vi "UHR-Fleezers Control (host) - Lorentz v2.vi"() -> ()   [LabVIEW 2014] (continued)
            n1300 = To Word Integer(number=w1984) -> (16bit integer=w1982:cluster{"Set 1":i16, "Set 2":i16})
          }
          frame True {
            n1301 = Unbundle By Name(w1992) -> ("Set 1"=w1991:dbl, "Set 2"=w1990:dbl)
            n1302 = Unbundle By Name(w1998) -> ("Set 1"=w1997:dbl, "Set 2"=w1996:dbl)
            n1303 = Unbundle By Name(w1995) -> ("Set 1"=w1994:bool, "Set 2"=w1993:bool)
            n1304 = Select(t=w1991, s=w1994, f=w1997) -> (s? t:f=w1989:dbl)
            n1305 = Select(t=w1990, s=w1993, f=w1996) -> (s? t:f=w1988:dbl)
            n1306 = Bundle By Name(cluster=w1998, "Set 1"=w1989, "Set 2"=w1988) -> (w1986:cluster{"Set 1":dbl, "Set 2":dbl})
            n1307 = local write "Setpoints (V)"(w1986) -> ()
            n1308 = Multiply(x=3276.7, y=w1986) -> (x*y=w1987:cluster{"Set 1":dbl, "Set 2":dbl})
            n1309 = To Word Integer(number=w1987) -> (16bit integer=w1999:cluster{"Set 1":i16, "Set 2":i16})
          }
        }
        n1310 = Unbundle By Name(w1971) -> ("Set 1"=w1970:i16, "Set 2"=w1969:i16)
        n1311 = xnode "Read/Write Control"("FPGA VI Reference In"=w1968, "error in"=w1967, "FB Setpoint Set 1"=w1970, "FB Setpoint Set 2"=w1969) -> ("error out"=w1966:errorcluster)  [unwired: 1 out]
      }
      event "+ phase (GI)", "- phase (GI)", "+ phase (GI) 2", "- phase (GI) 2", "+ phase (RI)", "- phase (RI)", "+ phase (Green FB)", "- phase (Green FB)", "- phase (BI AO)", "+ phase (BI AO)", "- phase (BI DO)", "+ phase (BI DO)": Value Change {
        n1312 = event-data() -> ()  [unwired: 7 out]
        n1313 = Or(x="+ phase (GI)", y="- phase (GI)") -> (x .or. y?=w2035:bool)
        n1314 = Negate(x="Phase adj. (GI)") -> (-x=w2040:i16)
        n1315 = Select(t=w2040, s="+ phase (GI)", f="Phase adj. (GI)") -> (s? t:f=w2039:i16)
        n1316 = Or(x="+ phase (GI) 2", y="- phase (GI) 2") -> (x .or. y?=w2026:bool)
        n1317 = Negate(x="Phase adj. (GI) 2") -> (-x=w2031:i16)
        n1318 = Select(t=w2031, s="+ phase (GI) 2", f="Phase adj. (GI) 2") -> (s? t:f=w2027:i16)
        n1319 = Negate(x="Phase adj. (RI)") -> (-x=w2025:i16)
        n1320 = Or(x="+ phase (RI)", y="- phase (RI)") -> (x .or. y?=w2021:bool)
        n1321 = Select(t=w2025, s="+ phase (RI)", f="Phase adj. (RI)") -> (s? t:f=w2020:i16)
        n1322 = Or(x="+ phase (Green FB)", y="- phase (Green FB)") -> (x .or. y?=w2014:bool)
        n1323 = Negate(x="Phase adj. (Green FB)") -> (-x=w2019:i16)
        n1324 = Select(t=w2019, s="+ phase (Green FB)", f="Phase adj. (Green FB)") -> (s? t:f=w2015:i16)
        n1325 = Negate(x="Phase adj. (BI AO)") -> (-x=w2013:i16)
        n1326 = Or(x="+ phase (BI AO)", y="- phase (BI AO)") -> (x .or. y?=w2003:bool)
        n1327 = Select(t=w2013, s="+ phase (BI AO)", f="Phase adj. (BI AO)") -> (s? t:f=w2005:i16)
        n1328 = Negate(x="Phase adj. (BI DO)") -> (-x=w2009:i16)
        n1329 = Or(x="+ phase (BI DO)", y="- phase (BI DO)") -> (x .or. y?=w2002:bool)
        n1330 = Select(t=w2009, s="+ phase (BI DO)", f="Phase adj. (BI DO)") -> (s? t:f=w2004:i16)
        n1331 = xnode "Read/Write Control"("FPGA VI Reference In"=w2001, "Phase count adjustment (GI)"=w2039, "Phase count adjustment (GI) 2"=w2027, "Phase count adjustment (RI)"=w2020, "Phase count adjustment (Green FB)"=w2015, "Phase count adjustment (BI AO)"=w2005, "Phase count adjustment (BI D)"=w2004) -> ("FPGA VI Reference Out"=w2037:T31, "error out"=w2038:errorcluster)  [unwired: 1 in]
        n1332 = xnode "Read/Write Control"("FPGA VI Reference In"=w2037, "error in"=w2038, "+ phase (GI)"=w2035, "+ phase (GI) 2"=w2026, "+ phase (RI)"=w2021, "+ phase (Green FB)"=w2014, "+ phase (BI AO)"=w2003, "+ phase (BI D)"=w2002) -> ("error out"=w2036:errorcluster)  [unwired: 1 out]
      }
      event "Green Laser ON/OFF", "Red Laser ON/OFF", "Blue Laser ON/OFF": Value Change {
        # "This loop shouldn't be initialized.  The main 'laser ON' settings should dominate and set the others."
        n1333 = event-data() -> ()  [unwired: 7 out]
        n1334 = property on="Red Laser ON" class="Bool (strict)"("Val(Sgnl)"="Red Laser ON/OFF") -> ()  [unwired: 2 in, 2 out]
        n1335 = property on="Blue Laser ON" class="Bool (strict)"("Val(Sgnl)"="Blue Laser ON/OFF") -> ()  [unwired: 2 in, 2 out]
        n1336 = property on="Green Laser ON" class="Bool (strict)"("Val(Sgnl)"="Green Laser ON/OFF") -> ()  [unwired: 2 in, 2 out]
      }
      event "Laser interlacing mode", "Green Laser ON", "Red Laser ON", "Blue Laser ON": Value Change {
        n1337 = event-data() -> ()  [unwired: 7 out]
        n1338 = local write "Green Laser ON/OFF"("Green Laser ON") -> ()
        n1339 = local write "Blue Laser ON/OFF"("Blue Laser ON") -> ()
        n1340 = local write "Red Laser ON/OFF"("Red Laser ON") -> ()
        n1341 = case shown="False" "Green Laser ON" {
          tunnel: "Laser interlacing mode" -> [_ w2101]
          tunnel: [enum32{"Laser ON", "Laser OFF", "Interlace"}."Laser OFF" ("Green laser mode") w2101] -> w2077
          tunnel: [FALSE w2097] -> w2076
          frame False {
          }
          frame True {
            n1342 = local read "Green FB On/Off"() -> (w2098:bool)
            n1343 = Equal?(x=w2101, y=enum32{"Laser ON", "Laser OFF", "Interlace"}."Interlace") -> (x = y?=w2099:bool)
            n1344 = And(x=w2099, y=w2098) -> (x .and. y?=w2097:bool)
          }
        }
        n1345 = case shown="True" "Red Laser ON" {
          tunnel: "Laser interlacing mode" -> [_ w2094]
          tunnel: [enum32{"Laser ON", "Laser OFF", "Interlace"}."Laser OFF" ("Green laser mode") w2094] -> w2073
          tunnel: [FALSE w2090] -> w2072
          frame False {
          }
          frame True {
            n1346 = local read "Red FB On/Off"() -> (w2091:bool)
            n1347 = Equal?(x=w2094, y=enum32{"Laser ON", "Laser OFF", "Interlace"}."Interlace") -> (x = y?=w2092:bool)
            n1348 = And(x=w2092, y=w2091) -> (x .and. y?=w2090:bool)
          }
        }
        n1349 = case shown="True" "Blue Laser ON" {
          tunnel: "Laser interlacing mode" -> [_ w2085]
          tunnel: [enum32{"Laser ON", "Laser OFF", "Interlace"}."Laser OFF" ("Green laser mode") w2085] -> w2069
          tunnel: [FALSE w2083] -> w2068
          frame False {
          }
          frame True {
            n1350 = local read "Blue FB On/Off"() -> (w2084:bool)
            n1351 = Equal?(x=w2085, y=enum32{"Laser ON", "Laser OFF", "Interlace"}."Interlace") -> (x = y?=w2086:bool)
            n1352 = And(x=w2086, y=w2084) -> (x .and. y?=w2083:bool)
          }
        }
        n1353 = xnode "Read/Write Control"("FPGA VI Reference In"=w2067, "Operating Mode"=w2077, "Operating Mode 2"=w2077, "Green FB On/Off"=w2076, "Red Laser Operating Mode"=w2073, "RI Operating Mode 2"=w2073, "Red FB On/Off"=w2072, "BI Operating Mode (AO)"=w2069, "Blue Laser Operating Mode (D)"=w2069, "Blue FB On/Off"=w2068) -> ("error out"=w2078:errorcluster)  [unwired: 1 in, 1 out]
        n1354 = local read "Red FB On/Off"() -> (w2050:bool)
        n1355 = local read "Green FB On/Off"() -> (w2052:bool)
        n1356 = local read "Green Laser ON"() -> (w2051:bool)
        n1357 = local read "Red Laser ON"() -> (w2049:bool)
        n1358 = And(x=w2050, y=w2049) -> (x .and. y?=w2055:bool)
        n1359 = And(x=w2052, y=w2051) -> (x .and. y?=w2061:bool)
        n1360 = local read "Red laser intensity (V)"() -> (w2054:dbl)
        n1361 = local read "Red FB Setpoint (mV)"() -> (w2053:dbl)
        n1362 = local read "Green FB Setpoint (mV)"() -> (w2064:dbl)
        n1363 = local read "Green laser intensity (V)"() -> (w2066:dbl)
        n1364 = Multiply(x=w2054, y=1000.0) -> (x*y=w2058:dbl)
        n1365 = Subtract(x=w2053, y=5.0) -> (x-y=w2057:dbl)
        n1366 = Multiply(x=w2066, y=1000.0) -> (x*y=w2063:dbl)
        n1367 = Subtract(x=w2064, y=5.0) -> (x-y=w2062:dbl)
        n1368 = Less Or Equal?(x=w2058, y=w2057) -> (x <= y?=w2056:bool)
        n1369 = Less Or Equal?(x=w2063, y=w2062) -> (x <= y?=w2060:bool)
        n1370 = And(x=w2055, y=w2056) -> (x .and. y?=w2045:bool)
        n1371 = And(x=w2061, y=w2060) -> (x .and. y?=w2046:bool)
        n1372 = Or(x=w2046, y=w2045) -> (x .or. y?=w2044:bool)
        n1373 = case shown="True" w2044 {
          frame False {
            n1374 = local write "Laser Intensity Low (bugs to fix)"(FALSE ("Laser Intensity Low")) -> ()
          }
          frame True {
            n1375 = local write "Laser Intensity Low (bugs to fix)"(TRUE ("Laser Intensity Low")) -> ()
          }
        }
      }
      event "Invert laser interlacing": Value Change {
        n1376 = event-data() -> ()  [unwired: 7 out]
        n1377 = xnode "Read/Write Control"("FPGA VI Reference In"=w2102, "Invert GI"="Invert laser interlacing", "Invert GI 2"="Invert laser interlacing", "Invert RI"="Invert laser interlacing", "Invert RI 2"="Invert laser interlacing", "Invert BI (AO)"="Invert laser interlacing", "Invert BI (D)"="Invert laser interlacing") -> ("error out"=w2104:errorcluster)  [unwired: 1 in, 1 out]
      }
      event "Green FB Setpoint (mV)", "Green FB Gains", "Green FB On/Off", "Green Intensity % (FB OFF)", "Green int current ON count adj": Value Change {
        n1378 = event-data() -> ()  [unwired: 7 out]
        n1379 = local read "Green FB Setpoint (mV)"() -> (w2124:dbl)
        n1380 = Multiply(x=w2124, y=3.2767) -> (x*y=w2123:dbl)
        n1381 = local read "Green Intensity % (FB OFF)"() -> (w2127:dbl)
        n1382 = Multiply(x=w2127, y=655.35) -> (x*y=w2128:dbl)
        n1383 = To Unsigned Word Integer(number=w2128) -> (unsigned 16bit integer=w2126:u16)
        n1384 = local read "Green int current ON count adj"() -> (w2130:u32)
        n1385 = local read "Laser interlacing mode"() -> (w2121:enum32{"Laser ON", "Laser OFF", "Interlace"})
        n1386 = local read "Green FB Gains"() -> (w2118:T11)
        n1387 = local read "Green Laser ON"() -> (w2122:bool)
        n1388 = local read "Green FB On/Off"() -> (w2131:bool)
        n1389 = Equal?(x=w2121, y=enum32{"Laser ON", "Laser OFF", "Interlace"}."Interlace") -> (x = y?=w2119:bool)
        n1390 = Unbundle By Name(w2118) -> ("proportional gain (Kc)"=w2117:i16, "integral gain (Kc*Ts/Ti)"=w2116:i16, "derivative gain (Kc*Td/Ts)"=w2115:i16)
        n1391 = Compound Arithmetic op=AND(w2119, w2131, w2122) -> (w2105:bool)
        n1392 = local read "Green FB Setpoint (mV)"() -> (w2109:dbl)
        n1393 = local read "Green laser intensity (V)"() -> (w2112:dbl)
        n1394 = xnode "Read/Write Control"("FPGA VI Reference In"=w2114, "Green FB Setpoint"=w2123, "Green FB On/Off"=w2105, "Current Out"=w2126, "Green int current ON count adj"=w2130, "P3"=w2117, "I3"=w2116, "D3"=w2115) -> ("error out"=w2132:errorcluster)  [unwired: 1 in, 1 out]
        n1395 = Multiply(x=w2112, y=1000.0) -> (x*y=w2108:dbl)
        n1396 = Subtract(x=w2109, y=5.0) -> (x-y=w2107:dbl)
        n1397 = Less Or Equal?(x=w2108, y=w2107) -> (x <= y?=w2106:bool)
        n1398 = And(x=w2105, y=w2106) -> (x .and. y?=w2113:bool)
        n1399 = case shown="True" w2113 {
          frame False {
            n1400 = local write "Laser Intensity Low (bugs to fix)"(FALSE ("Laser Intensity Low")) -> ()
          }
          frame True {
            n1401 = local write "Laser Intensity Low (bugs to fix)"(TRUE ("Laser Intensity Low")) -> ()
          }
        }
      }
      event "Blue FB Setpoint (mV)", "Blue FB Gains", "Blue FB On/Off", "Blue Intensity % (FB OFF)", "Blue int AO ON count adjust": Value Change {
        # "Triggers blue laser serial command"
        # "16 bit analog out"
        n1402 = event-data() -> ()  [unwired: 7 out]
        n1403 = Multiply(x="Blue FB Setpoint (mV)", y=3.2767) -> (x*y=w2152:dbl)
        n1404 = Multiply(x="Blue Intensity % (FB OFF)", y=0.8) -> (x*y=w2135:dbl)
        n1405 = Number To Decimal String(number=w2135) -> (decimal integer string=w2136:string)  [unwired: 1 in]
        n1406 = Multiply(x="Blue Intensity % (FB OFF)", y=655.35) -> (x*y=w2155:dbl)
        n1407 = local write "Blue Laser Power (mW)\n(Constant Power Mode)"(w2136) -> ()
        n1408 = To Unsigned Word Integer(number=w2155) -> (unsigned 16bit integer=w2154:u16)
        n1409 = local read "Laser interlacing mode"() -> (w2150:enum32{"Laser ON", "Laser OFF", "Interlace"})
        n1410 = Unbundle By Name("Blue FB Gains") -> ("proportional gain (Kc)"=w2147:i16, "integral gain (Kc*Ts/Ti)"=w2146:i16, "derivative gain (Kc*Td/Ts)"=w2145:i16)
        n1411 = local read "Blue Laser ON"() -> (w2140:bool)
        n1412 = Equal?(x=w2150, y=enum32{"Laser ON", "Laser OFF", "Interlace"}."Interlace") -> (x = y?=w2148:bool)
        n1413 = Compound Arithmetic op=AND(w2148, "Blue FB On/Off", w2140) -> (w2151:bool)
        n1414 = xnode "Read/Write Control"("FPGA VI Reference In"=w2139, "Blue FB Setpoint"=w2152, "Blue FB On/Off"=w2151, "BI Current Out"=w2154, "Blue current ON count adj (AO)"="Blue int AO ON count adjust", "P5"=w2147, "I5"=w2146, "D5"=w2145) -> ("error out"=w2157:errorcluster)  [unwired: 1 in, 1 out]
      }
      event "Red FB Setpoint (mV)", "Red FB Gains", "Red FB On/Off", "Red Intensity % (FB OFF)": Value Change {
        n1415 = event-data() -> ()  [unwired: 7 out]
        n1416 = local read "Red FB Setpoint (mV)"() -> (w2178:dbl)
        n1417 = Multiply(x=w2178, y=3.2767) -> (x*y=w2177:dbl)
        n1418 = local read "Red Intensity % (FB OFF)"() -> (w2168:dbl)
        n1419 = Multiply(x=w2168, y=655.35) -> (x*y=w2181:dbl)
        n1420 = To Unsigned Word Integer(number=w2181) -> (unsigned 16bit integer=w2180:u16)
        n1421 = local read "Laser interlacing mode"() -> (w2175:enum32{"Laser ON", "Laser OFF", "Interlace"})
        n1422 = local read "Red FB Gains"() -> (w2172:T11)
        n1423 = local read "Red Laser ON"() -> (w2176:bool)
        n1424 = local read "Red FB On/Off"() -> (w2183:bool)
        n1425 = Equal?(x=w2175, y=enum32{"Laser ON", "Laser OFF", "Interlace"}."Interlace") -> (x = y?=w2173:bool)
        n1426 = Unbundle By Name(w2172) -> ("proportional gain (Kc)"=w2171:i16, "integral gain (Kc*Ts/Ti)"=w2170:i16, "derivative gain (Kc*Td/Ts)"=w2169:i16)
        n1427 = Compound Arithmetic op=AND(w2173, w2183, w2176) -> (w2160:bool)
        n1428 = local read "Red laser intensity (V)"() -> (w2159:dbl)
        n1429 = local read "Red FB Setpoint (mV)"() -> (w2158:dbl)
        n1430 = xnode "Read/Write Control"("FPGA VI Reference In"=w2167, "Red FB Setpoint"=w2177, "Red FB On/Off"=w2160, "RI Current Out"=w2180, "P4"=w2171, "I4"=w2170, "D4"=w2169) -> ("error out"=w2184:errorcluster)  [unwired: 1 in, 1 out]
        n1431 = Multiply(x=w2159, y=1000.0) -> (x*y=w2164:dbl)
        n1432 = Subtract(x=w2158, y=5.0) -> (x-y=w2163:dbl)
        n1433 = Less Or Equal?(x=w2164, y=w2163) -> (x <= y?=w2162:bool)
        n1434 = And(x=w2160, y=w2162) -> (x .and. y?=w2161:bool)
        n1435 = case shown="False" w2161 {
          frame False {
            n1436 = local write "Laser Intensity Low (bugs to fix)"(FALSE ("Laser Intensity Low")) -> ()
          }
          frame True {
            n1437 = local write "Laser Intensity Low (bugs to fix)"(TRUE ("Laser Intensity Low")) -> ()
          }
        }
      }
      event "+ phase (APD 1 Gate)", "- phase (APD 1 Gate)", "+ phase (APD 2 Gate)", "- phase (APD 2 Gate)", "+ phase (APD 3 Gate)", "- phase (APD 3 Gate)", "+ phase (APD Acq)", "- phase (APD Acq)": Value Change {
        n1438 = event-data() -> ()  [unwired: 7 out]
        n1439 = local read "Phase Adj. (APD 1 Gate)"() -> (w2207:i16)
        n1440 = Or(x="- phase (APD 1 Gate)", y="+ phase (APD 1 Gate)") -> (x .or. y?=w2209:bool)
        n1441 = Negate(x=w2207) -> (-x=w2214:i16)
        n1442 = Select(t=w2214, s="+ phase (APD 1 Gate)", f=w2207) -> (s? t:f=w2213:i16)
        n1443 = local read "Phase Adj. (APD 2 Gate)"() -> (w2204:i16)
        n1444 = Or(x="- phase (APD 2 Gate)", y="+ phase (APD 2 Gate)") -> (x .or. y?=w2202:bool)
        n1445 = Negate(x=w2204) -> (-x=w2206:i16)
        n1446 = Select(t=w2206, s="+ phase (APD 2 Gate)", f=w2204) -> (s? t:f=w2203:i16)
        n1447 = Negate(x="Phase Adj. (APD 3 Gate)") -> (-x=w2201:i16)
        n1448 = Or(x="- phase (APD 3 Gate)", y="+ phase (APD 3 Gate)") -> (x .or. y?=w2197:bool)
        n1449 = Select(t=w2201, s="+ phase (APD 3 Gate)", f="Phase Adj. (APD 3 Gate)") -> (s? t:f=w2198:i16)
        n1450 = local read "Phase Adj. (APD Acq)"() -> (w2195:i16)
        n1451 = Or(x="- phase (APD Acq)", y="+ phase (APD Acq)") -> (x .or. y?=w2193:bool)
        n1452 = Negate(x=w2195) -> (-x=w2196:i16)
        n1453 = Select(t=w2196, s="+ phase (APD Acq)", f=w2195) -> (s? t:f=w2194:i16)
        n1454 = xnode "Read/Write Control"("FPGA VI Reference In"=w2187, "Phase count adjustment (APD 1 Gate)"=w2213, "Phase count adjustment (APD 2 Gate)"=w2203, "Phase count adjustment (APD 3 Gate)"=w2198, "Phase Count Adjustment (APD Acq)"=w2194) -> ("FPGA VI Reference Out"=w2211:T31, "error out"=w2212:errorcluster)  [unwired: 1 in]
        n1455 = xnode "Read/Write Control"("FPGA VI Reference In"=w2211, "error in"=w2212, "+ phase (APD 1 Gate)"=w2209, "+ phase (APD 2 Gate)"=w2202, "+ phase (APD 3 Gate)"=w2197, "+ phase (APD Acq)"=w2193) -> ("error out"=w2210:errorcluster)  [unwired: 1 out]
      }
      event "Invert APD Gate", "APD Gate ON Count", "APD Gate OFF Count", "APD Gate", "APD Integration Time (s)", "APD AO Scale Factor", "Duty Frequency (ON 1/N cycles)", "Interlace ON count", "Interlace OFF count": Value Change {
        n1456 = event-data() -> ()  [unwired: 7 out]
        n1457 = Add(x="Interlace ON count", y="Interlace OFF count") -> (x+y=w2221:u16)
        n1458 = Add(x="APD Gate ON Count", y="APD Gate OFF Count") -> (x+y=w2232:u16)
        n1459 = Multiply(x="Duty Frequency (ON 1/N cycles)", y=w2221) -> (x*y=w2217:u16)
        "Green AI Count" <- w2217
        "Red AI Count" <- w2217
        "Blue AI Count" <- w2217
        n1460 = Subtract(x=w2217, y="Interlace ON count") -> (x-y=w2220:u16)
        n1461 = Multiply(x=w2232, y="Duty Frequency (ON 1/N cycles)") -> (x*y=w2231:u16)
        n1462 = Subtract(x=w2231, y="APD Gate ON Count") -> (x-y=w2230:u16)
        n1463 = local read "DMA Update Period (s)"() -> (w2233:dbl)
        n1464 = Multiply(x="APD Integration Time (s)", y=40000000.0) -> (x*y=w2237:dbl)
        n1465 = Reciprocal(x="APD Integration Time (s)") -> (1/x=→"APD Acq Rate (Hz)":dbl)
        n1466 = To Unsigned Long Integer(number=w2237) -> (unsigned 32bit integer=w2223:u32)
        "APD Int. Count" <- w2223
        n1467 = local read "Number of APDs"() -> (w2216:u8)
        n1468 = Divide(x=w2233, y="APD Integration Time (s)") -> (x/y=w2235:dbl)
        n1469 = Multiply(x=w2216, y=w2235) -> (x*y=w2234:dbl)
        n1470 = local write "APD Samples/FIFO Acq."(w2235) -> ()
        n1471 = local write "APD Elements/DMA read"(w2234) -> ()
        n1472 = xnode "Read/Write Control"("FPGA VI Reference In"=w2215, "Invert APD Gate"="Invert APD Gate", "APD Gate ON Count"="APD Gate ON Count", "APD Gate OFF Count"=w2230, "APD Acq Rate Count"=w2223, "APD Gate Operating Mode"="APD Gate", "APD AO scale factor"="APD AO Scale Factor", "Green interlace ON count"="Interlace ON count", "Green interlace OFF count"=w2220, "Green interlace ON count 2"="Interlace ON count", "Green interlace OFF count 2"=w2220, "Green FB Count"=w2217, "Red interlace ON count"="Interlace ON count", "Red interlace OFF count"="Interlace OFF count", "Blue ON count (AO)"="Interlace ON count", "Blue OFF count (AO)"="Interlace OFF count", "Blue interlace OFF count (D)"="Interlace OFF count", "Blue interlace ON count (D)"="Interlace ON count") -> ("error out"=w2239:errorcluster)  [unwired: 1 in, 1 out]
      }
      event "Neg. TTrig FPGA": Value Change {
        n1473 = event-data() -> ()  [unwired: 7 out]
        n1474 = xnode "Read/Write Control"("FPGA VI Reference In"=w2240, "TTrig Negate Pos"="Neg. TTrig FPGA") -> ()  [unwired: 1 in, 2 out]
      }
      event "Test ttrig": Value Change {
        n1475 = event-data() -> ()  [unwired: 7 out]
        n1476 = xnode "Read/Write Control"("FPGA VI Reference In"=w2242, "TTrig?"=TRUE) -> ("error out"=w2244:errorcluster)  [unwired: 1 in, 1 out]
      }
      event "Number of F/B Scans (AOD)", "Scan Speed (nm/s)", "Scan BD", "Initial delta (MHz)", "Step Size (nm)", "Scan Range (nm)": Value Change {
        w2308 = 123.0  # AOM cal (nm/MHz)
        n1477 = event-data() -> ()  [unwired: 7 out]
        n1478 = local read "BD 1 Frequency 1 (MHz)"() -> (w2291:dbl)
        n1479 = local read "AOM X Cal (nm/MHz)"() -> (w2283:dbl)
        n1480 = local read "X RF Frequency Limits (MHz)"() -> (w2295:T20)
        n1481 = local read "Y RF Frequency Limits (MHz)"() -> (w2292:T20)
        n1482 = local read "BD 2 Frequency 1 (MHz)"() -> (w2297:dbl)
        n1483 = Negate(x="Scan Range (nm)") -> (-x=w2261:dbl)
        n1484 = Divide(x=w2261, y=w2283) -> (x/y=w2265:dbl)
        n1485 = Select(t=w2295, s="Scan BD", f=w2292) -> (s? t:f=w2294:T20)
        n1486 = Select(t=w2291, s="Scan BD", f=w2297) -> (s? t:f=w2296:dbl)
        n1487 = Unbundle By Name(w2294) -> ("Maximum"=w2303:dbl, "Minimum"=w2302:dbl)
        n1488 = Add(x=w2265, y=w2296) -> (x+y=w2300:dbl)
        n1489 = Divide(x=w2261, y="Step Size (nm)") -> (x/y=w2280:dbl)
        n1490 = Divide(x="Step Size (nm)", y=w2283) -> (x/y=w2289:dbl)
        n1491 = Absolute Value(x=w2280) -> (abs(x)=w2264:dbl)
        n1492 = Sign(1:w2261) -> (0:w2262:dbl)
        n1493 = In Range and Coerce(upper limit=w2303, x=w2300, lower limit=w2302) -> (coerced(x)=w2299:dbl, In Range?=w2301:bool)
        n1494 = To Unsigned Quad Integer(1:w2264) -> (0:w2279:u64)
        "Scan steps (AOD)" <- w2279
        n1495 = call "IR AOM freq to word.vi"("Frequency In (MHz)"=w2289) -> ("Frequency Word Out (double)"=w2286:dbl)
        n1496 = Multiply(x=w2262, y=w2286) -> (x*y=w2263:dbl)
        n1497 = Subtract(x=w2300, y=w2299) -> (x-y=w2298:dbl)
        n1498 = To Quad Integer(1:w2263) -> (0:w2285:i64)
        "Incr. int (AOD)" <- w2285
        n1499 = Subtract(x=w2265, y=w2298) -> (x-y=w2284:dbl)
        "Scan Range (MHz)" <- w2284
        n1500 = Select(t=w2265, s=w2301, f=w2284) -> (s? t:f=w2304:dbl)
        n1501 = Multiply(x=w2284, y=w2283) -> (x*y=w2282:dbl)
        n1502 = Decrement(x=w2279) -> (x-1=w2332:u64)
        n1503 = Negate(x=w2282) -> (-x=w2278:dbl)
        n1504 = local write "Scan Range (nm)"(w2278) -> ()
        n1505 = Divide(x=w2304, y=w2332) -> (x/y=w2288:dbl)
        "Scan Increment (MHz)" <- w2288
        n1506 = call "IR AOM freq to word.vi"("Frequency In (MHz)"=w2288) -> ("Frequency Word Out (double)"=w2287:dbl)
        n1507 = Divide(x="Step Size (nm)", y="Scan Speed (nm/s)") -> (x/y=w2275:dbl)
        n1508 = To Quad Integer(1:w2287) -> ()  [unwired: 1 out]
        n1509 = local read "Number Interlace Sets"() -> (w2259:u8)
        n1510 = local read "AI Count (ticks)"() -> (w2260:u16)
        n1511 = local read "Total Counts (ticks)"() -> (w2258:u16)
        n1512 = local read "# Samples/trap"() -> (w2290:u32)
        n1513 = Multiply(x=w2260, y=w2259) -> (x*y=w2257:u16)
        n1514 = Divide(x=w2258, y=w2257) -> (x/y=w2256:dbl)
        n1515 = Select(t=w2291, s="Scan BD", f=w2297) -> (s? t:f=w2329:dbl)
        "Initial freq. (MHz)" <- w2329
        n1516 = Add(x=w2304, y=w2329) -> (x+y=→"Final freq. (MHz)":dbl)
        n1517 = Divide(x=w2258, y=40000000.0) -> (x/y=w2274:dbl)
        n1518 = Divide(x=w2275, y=w2274) -> (x/y=w2273:dbl)
        n1519 = To Unsigned Quad Integer(1:w2273) -> (0:w2248:u64)
        n1520 = Quotient & Remainder(x=w2248, y=u64 2) -> (x-y*floor(x/y)=w2252:u64)  [unwired: 1 out]
        n1521 = Equal?(x=w2252, y=u64 0) -> (x = y?=w2250:bool)
        n1522 = Decrement(x=w2248) -> (x-1=w2249:u64)
        n1523 = Select(t=w2248, s=w2250, f=w2249) -> (s? t:f=w2247:u64)
        "Cycles/step (AOD)" <- w2247
        n1524 = xnode "Read/Write Control"("FPGA VI Reference In"=w2246, "Scan steps"=w2279, "Number of scans"="Number of F/B Scans (AOD)", "Cycles per step"=w2247, "Scan freq.  increment"=w2285, "Scan BD"="Scan BD") -> ("error out"=w2338:errorcluster)  [unwired: 1 in, 1 out]
        n1525 = Multiply(x=w2279, y=w2247) -> (x*y=w2333:u64)
        n1526 = Multiply(x=w2333, y=u64 2) -> (x*y=w2255:u64)
        n1527 = Multiply(x=w2256, y=w2255) -> (x*y=w2254:dbl)
        "Data points/scan (f/b)" <- w2254
        n1528 = Multiply(x=w2254, y="Number of F/B Scans (AOD)") -> (x*y=w2336:dbl)
        "Data points/scans" <- w2336
        n1529 = Divide(x=w2336, y=w2290) -> (x/y=→"N sets should be saved":dbl)
        n1530 = Multiply(x=w2333, y=w2274) -> (x*y=w2272:dbl)
        "Time/Scan (s) (AOD)" <- w2272
        n1531 = Select(t=w2304, s="Scan BD", f=0.0) -> (s? t:f=w2330:dbl)
        n1532 = Select(t=0.0, s="Scan BD", f=w2304) -> (s? t:f=w2326:dbl)
        n1533 = local read "BD 2 Frequency 2 (MHz)"() -> (w2322:dbl)
        n1534 = local read "BD 1 Frequency 2 (MHz)"() -> (w2325:dbl)
        n1535 = Add(x=w2326, y=w2297) -> (x+y=w2323:dbl)
        n1536 = Add(x=w2291, y=w2330) -> (x+y=w2324:dbl)
        n1537 = Multiply(x=w2272, y=2.0) -> (x*y=w2271:dbl)
        n1538 = Multiply(x=w2271, y="Number of F/B Scans (AOD)") -> (x*y=w2268:dbl)
        n1539 = Divide(x=w2268, y=60.0) -> (x/y=→"Time to Finish All (min)":dbl)
        n1540 = Add(x="Trap 2 Bead Size (nm)", y="Trap 1 Bead Size (nm)") -> (x+y=w2312:dbl)
        n1541 = Divide(x=w2312, y=2.0) -> (x/y=w2306:dbl)
        n1542 = local read "Initial delta (MHz)"() -> (w2309:dbl)
        n1543 = Subtract(x=w2323, y=w2322) -> (x-y=w2320:dbl)
        n1544 = Subtract(x=w2324, y=w2325) -> (x-y=w2321:dbl)
        n1545 = Square(x=w2320) -> (x^2=w2319:dbl)
        n1546 = Square(x=w2321) -> (x^2=w2318:dbl)
        n1547 = Add(x=w2318, y=w2319) -> (x+y=w2317:dbl)
        n1548 = Square Root(x=w2317) -> (sqrt(x)=w2316:dbl)
        "Final delta (MHz)" <- w2316
        n1549 = Multiply(x=w2308, y=w2316) -> (x*y=w2315:dbl)
        n1550 = Multiply(x=w2309, y=w2308) -> (x*y=w2307:dbl)
        n1551 = Subtract(x=w2307, y=w2306) -> (x-y=→"Initial sep (nm)":dbl)
        n1552 = Subtract(x=w2315, y=w2306) -> (x-y=→"Final sep (nm)":dbl)
      }
      event "Freq or Amp switch first", "Swap F1 and F2", "Freq switch delay", "Amp switch delay": Value Change {
        n1553 = event-data() -> ()  [unwired: 7 out]
        n1554 = local read "Amp switch delay"() -> (w2340:u16)
        n1555 = local read "Swap F1 and F2"() -> (w2341:bool)
        n1556 = xnode "Read/Write Control"("FPGA VI Reference In"=w2339, "Swap F1 and F2"=w2341, "Amp switch delay"=w2340) -> ("error out"=w2342:errorcluster)  [unwired: 1 in, 1 out]
      }
      event "Scan steps (MCL)", "Number of scans (MCL)", "Scan Range (V)\n(of steps)", "2D or 1D Scan", "N APD Samp/step", "Fast Scan Dir", "Continuous MCL Scanning", "Scan lines (y)": Value Change {
        w2345 = 32767.0 ("y")
        n1557 = event-data() -> ()  [unwired: 7 out]
        n1558 = Select(t="Scan lines (y)", s="2D or 1D Scan", f="Number of scans (MCL)") -> (s? t:f=w2350:u64)
        n1559 = Decrement(x="Scan steps (MCL)") -> (x-1=w2366:u64)
        n1560 = Divide(x="Scan Range (V)\n(of steps)", y=w2366) -> (x/y=w2365:dbl)
        "Desired Scan Incr (V)" <- w2365
        n1561 = local read "APD Integration Time (s)"() -> (w2358:dbl)
        n1562 = Multiply(x=w2365, y=w2345) -> (x*y=w2374:dbl)
        n1563 = Divide(x=w2374, y=10.0) -> (x/y=w2364:dbl)
        "Desired incr (int)" <- w2364
        n1564 = local read "Update Count (MCL)"() -> (w2370:u32)
        n1565 = Round Toward -Infinity(1:w2364) -> (0:w2373:dbl)
        n1566 = To Word Integer(number=w2373) -> (16bit integer=w2348:i16)
        "Actual Incr. int (MCL)" <- w2348
        n1567 = Multiply(x=w2358, y=40000000.0) -> (x*y=w2371:dbl)
        n1568 = Divide(x=w2371, y=w2370) -> (x/y=w2369:dbl)
        n1569 = Multiply(x=i16 10, y=w2348) -> (x*y=w2346:i16)
        n1570 = Multiply(x="N APD Samp/step", y=w2369) -> (x*y=w2368:dbl)
        "Cycles/step (MCL)" <- w2368
        n1571 = Divide(x=w2346, y=w2345) -> (x/y=→"Actual MCL Inc (V)":dbl)
        n1572 = Multiply(x="N APD Samp/step", y="Scan steps (MCL)") -> (x*y=w2360:dbl)
        n1573 = local read "APD Samples/FIFO Acq."() -> (w2357:dbl)
        n1574 = Multiply(x=w2360, y=u64 2) -> (x*y=w2359:dbl)
        "Data points/scan (f+b)" <- w2359
        n1575 = Multiply(x=w2359, y=w2350) -> (x*y=w2377:dbl)
        "Data points/scans (MCL)" <- w2377
        n1576 = Multiply(x=w2358, y=w2359) -> (x*y=w2351:dbl)
        "Time/f+b scan (s) (MCL)" <- w2351
        n1577 = Divide(x=w2377, y=w2357) -> (x/y=→"N sets should be saved (MCL)":dbl)
        n1578 = Multiply(x=w2351, y=w2350) -> (x*y=→"Total Time (s)":dbl)
        n1579 = Not(x="Fast Scan Dir") -> (.not. x?=w2355:bool)
        n1580 = xnode "Read/Write Control"("FPGA VI Reference In"=w2343, "Scan steps (MCL)"="Scan steps (MCL)", "Number of scans (MCL)"=w2350, "Cycles per step (MCL)"=w2368, "Scan freq.  increment (MCL)"=w2348, "1D or 2D Scan?"="2D or 1D Scan", "MCL Scan Axis"=w2355, "Cont. Scan (MCL)"="Continuous MCL Scanning") -> ("error out"=w2379:errorcluster)  [unwired: 1 in, 1 out]
      }
      event "Read Cal": Value Change {
        w2418 = 1000.0 ("y")
        w2401 = T41."big-endian, network order" ("byte order (0:big-endian, network order)")
        w2402 = -1 ("count (1)")
        n1581 = event-data() -> ()  [unwired: 7 out]
        n1582 = local read "Save file name"() -> (w2434:path)
        n1583 = local write "Read Cal"(FALSE ("Read Cal")) -> ()
        n1584 = Strip Path(path=w2434) -> (stripped path=w2433:path)  [unwired: 1 out]
        n1585 = Path To String(path=w2433) -> (string=w2410:string)
        n1586 = Concatenate Strings(w2410, "\\current.cal" ("string")) -> (w2431:string)
        n1587 = Concatenate Strings(w2410, "\\current.off" ("string")) -> (w2408:string)
        n1588 = String To Path(string=w2431) -> (path=w2430:path)
        n1589 = String To Path(string=w2408) -> (path=w2405:path)
        n1590 = Open/Create/Replace File(file path (use dialog)=w2430, operation (0:open)=T40."open", access (0:read/write)=enum16{"read/write", "read-only", "write-only"}."read-only") -> (refnum out=w2437:refnum<file>, error out=w2426:errorcluster)  [unwired: 1 in, 3 out]
        n1591 = Open/Create/Replace File(file path (use dialog)=w2405, operation (0:open)=T40."open", access (0:read/write)=enum16{"read/write", "read-only", "write-only"}."read-only") -> (refnum out=w2404:refnum<file>)  [unwired: 1 in, 4 out]
        n1592 = Deny Access(4:w2426, 7:w2437) -> (0:w2425:errorcluster, 3:w2429:refnum<file>)  [unwired: 1 out]
        n1593 = Deny Access(7:w2404) -> (3:w2403:refnum<file>)  [unwired: 1 in, 2 out]
        n1594 = Read from Binary File(5:0.0, 8:w2425, 9:w2401, 10:w2402, 11:w2429) -> (0:w2424:errorcluster, 2:w2422:dbl[], 3:w2427:refnum<file>)  [unwired: 2 out]
        n1595 = Array To Cluster(array=w2422) -> (cluster=w2421:T43)
        n1596 = Unbundle(w2421) -> ("[0]"=w2389:dbl, "[1]"=w2387:dbl, "[2]"=w2388:dbl, "[3]"=w2386:dbl, "[4]"=w2420:dbl, "[5]"=w2419:dbl)
        n1597 = Close File(refnum=w2427, error in=w2424) -> (error out=→"Read cal error":errorcluster)  [unwired: 1 out]
        n1598 = Multiply(x=w2420, y=w2418) -> (x*y=w2415:dbl)
        n1599 = Multiply(x=w2419, y=w2418) -> (x*y=w2411:dbl)
        n1600 = Read from Binary File(5:0.0, 9:w2401, 10:w2402, 11:w2403) -> (2:w2397:dbl[], 3:w2395:refnum<file>)  [unwired: 1 in, 3 out]
        n1601 = Close File(refnum=w2395) -> ()  [unwired: 1 in, 2 out]
        n1602 = Bundle By Name(cluster="T1 calibration", "T1 alpha_x (nm/V)"=w2389, "T1 offset_x (mV)"=w2415, "T1 kappa_x (pN/nm)"=w2388) -> (w2414:T6)
        n1603 = Array Subset(array=w2397, index=1) -> (w2394:dbl[])  [unwired: 1 in]
        n1604 = Bundle By Name(cluster="T2 calibration", "T2 alpha_x (nm/V)"=w2387, "T2 offset_x (mV)"=w2411, "T2 kappa_x (pN/nm)"=w2386) -> (w2412:T5)
        n1605 = Index Array(array=w2397, index=0) -> (element=→"Offset file step size":dbl)
        n1606 = local write "T1 calibration"(w2414) -> ()
        n1607 = local write "T2 calibration"(w2412) -> ()
        n1608 = Decimate 1D Array(w2394) -> (w2384:dbl[], w2383:dbl[])  [unwired: 1 out]
        n1609 = Multiply(x=w2389, y=w2388) -> (x*y=w2390:dbl)
        n1610 = Multiply(x=w2387, y=w2386) -> (x*y=w2391:dbl)
        n1611 = Divide(x=w2391, y=w2390) -> (x/y=w2382:dbl)
        n1612 = property on="B factor" class="DigNum (strict)"("Val(Sgnl)"=w2382) -> ()  [unwired: 2 in, 2 out]
        n1613 = Bundle By Name(cluster="Offset Values", "Trap 1X offset"=w2384, "Trap 2X offset"=w2383) -> (w2392:T17)
        n1614 = Multiply(x=w2383, y=w2382) -> (x*y=w2385:dbl[])
        n1615 = local write "Offset Values"(w2392) -> ()
        n1616 = Subtract(x=w2384, y=w2385) -> (x-y=w2380:dbl[])
        n1617 = case shown="True" "Auto read offset correction" {
          tunnel: w2380 -> [_ w2438]
          frame False {
          }
          frame True {
            n1618 = property on="Setpoint offset\ncorrection values" class="Arr (strict)"("Val(Sgnl)"=w2438) -> ()  [unwired: 2 in, 2 out]
          }
        }
      }
      event "Abort MCL Scan": Value Change {
        n1619 = event-data() -> ()  [unwired: 7 out]
        n1620 = local write "MCL Scanning"(FALSE ("MCL Scanning")) -> ()
        n1621 = xnode "Read/Write Control"("FPGA VI Reference In"=w2439, "Abort scan (MCL)"="Abort MCL Scan") -> ("error out"=w2442:errorcluster)  [unwired: 1 in, 1 out]
      }
      event "Update Count (MCL)": Value Change {
        n1622 = event-data() -> ()  [unwired: 7 out]
        n1623 = xnode "Read/Write Control"("FPGA VI Reference In"=w2443, "MCL count"="Update Count (MCL)") -> ("error out"=w2445:errorcluster)  [unwired: 1 in, 1 out]
      }
      event "+ phase (MCL)", "- phase (MCL)": Value Change {
        n1624 = event-data() -> ()  [unwired: 7 out]
        n1625 = Or(x="- phase (MCL)", y="+ phase (MCL)") -> (x .or. y?=w2449:bool)
        n1626 = Negate(x="Phase adjust (MCL)") -> (-x=w2455:i16)
        n1627 = Select(t=w2455, s="+ phase (MCL)", f="Phase adjust (MCL)") -> (s? t:f=w2453:i16)
        n1628 = xnode "Read/Write Control"("FPGA VI Reference In"=w2446, "Phase count adjustment (MCL)"=w2453) -> ("FPGA VI Reference Out"=w2450:T31, "error out"=w2451:errorcluster)  [unwired: 1 in]
        n1629 = xnode "Read/Write Control"("FPGA VI Reference In"=w2450, "error in"=w2451, "+ phase (MCL)"=w2449) -> ("error out"=w2448:errorcluster)  [unwired: 1 out]
      }
      event "Abort AOD Scan": Value Change {
        n1630 = event-data() -> ()  [unwired: 7 out]
        n1631 = xnode "Read/Write Control"("FPGA VI Reference In"=w2456, "Abort scan"="Abort AOD Scan") -> ("error out"=w2458:errorcluster)  [unwired: 1 in, 1 out]
      }
      event "Continuous AOD Scanning": Value Change {
        n1632 = event-data() -> ()  [unwired: 7 out]
        n1633 = xnode "Read/Write Control"("FPGA VI Reference In"=w2459, "Cont. Scan"="Continuous AOD Scanning") -> ("error out"=w2461:errorcluster)  [unwired: 1 in, 1 out]
      }
      event "Index": Value Change {
        n1634 = event-data() -> ()  [unwired: 7 out]
        n1635 = call "Create new save file.vi"("Insert"="", "Ext"=".dat" ("string"), "Index In"="Index") -> ("Path Out"=→"Save file name":path, "Index Out"=w2462:dbl)
        "Save index" <- w2462
        n1636 = local write "Index"(w2462) -> ()
      }
      event "AO1", "AO2": Value Change {
        w2476 = 10.0 ("y")
        w2475 = 32767.0 ("y")
        n1637 = event-data() -> ()  [unwired: 7 out]
        n1638 = local read "AO2"() -> (w2474:dbl)
        n1639 = local read "AO1"() -> (w2471:dbl)
        n1640 = Multiply(x=w2471, y=w2475) -> (x*y=w2470:dbl)
        n1641 = Multiply(x=w2474, y=w2475) -> (x*y=w2473:dbl)
        n1642 = Divide(x=w2470, y=w2476) -> (x/y=w2469:dbl)
        n1643 = Divide(x=w2473, y=w2476) -> (x/y=w2472:dbl)
        n1644 = To Word Integer(number=w2469) -> (16bit integer=w2477:i16)
        n1645 = To Word Integer(number=w2472) -> (16bit integer=w2478:i16)
        n1646 = xnode "Read/Write Control"("FPGA VI Reference In"=w2467, "AO1"=w2477, "AO2"=w2478) -> ("error out"=w2468:errorcluster)  [unwired: 1 in, 1 out]
      }
      event "Inject Pump 1": Value Change {
        n1647 = event-data() -> ()  [unwired: 7 out]
        n1648 = disable-structure shown="Disabled" {
          disable-tunnel: w2479 -> [w2480 _]
          frame Disabled {
            n1649 = local read "Use Harvard pumps\nfor beads (else Chemyx)"() -> (w2481:bool)
            n1650 = case shown="True" w2481 {
              tunnel: "Inject Pump 1" -> [w2485 w2526]
              tunnel: w2480 -> [_ w2527]
              frame False {
                n1651 = local read "Pump write delay (ms)"() -> (w2484:dbl)
                n1652 = local read "Chemyx Syringe Pump Serial Port"() -> (w2483:refnum<visa-resource-name>)
                n1653 = case shown="True" w2485 {
                  tunnel: w2484 -> [w2491 w2505]
                  tunnel: w2483 -> [w2488 w2504]
                  frame False {
                    n1654 = flat-sequence {
                      tunnel: w2488 -> [w2492]
                      tunnel: [w2492] -> w2489
                      tunnel: w2491 -> [_]
                      tunnel: [w2495] -> w2490
                      tunnel: w2489 -> [w2495]
                      tunnel: w2490 -> [w2496]
                      tunnel: [w2496] -> w2486
                      tunnel: [w2498] -> w2487
                      tunnel: w2486 -> [w2498]
                      tunnel: w2487 -> [w2500]
                      frame #0 {
                        n1655 = call "Write to pump.vi"("string"="enter pump1", "VISA resource name"=w2492) -> ()  [unwired: 1 out]
                      }
                      frame #1 {
                        n1656 = Wait (ms)(milliseconds to wait="Pump pause delay (ms)") -> ()  [unwired: 1 out]
                      }
                      frame #2 {
                        n1657 = call "Write to pump.vi"("string"="stop", "VISA resource name"=w2496) -> ()  [unwired: 1 out]
                      }
                      frame #3 {
                        n1658 = Wait (ms)(milliseconds to wait=u32 500) -> ()  [unwired: 1 out]
                      }
                      frame #4 {
                        n1659 = call "Write to pump.vi"("string"="stop", "VISA resource name"=w2500) -> ()  [unwired: 1 out]
                      }
                    }
                  }
                  frame True {
                    n1660 = flat-sequence {
                      tunnel: w2504 -> [w2514]
                      tunnel: w2505 -> [w2509]
                      tunnel: w2505 -> [w2516]
                      tunnel: w2504 -> [w2517]
                      tunnel: [w2517] -> w2502
                      tunnel: [w2519] -> w2503
                      tunnel: w2502 -> [w2519]
                      tunnel: w2503 -> [w2521]
                      frame #0 {
                        n1661 = local read "All Pump Parameters"() -> (w2508:T7)
                        n1662 = Unbundle By Name(w2508) -> ("Pump 1"=w2515:T44)
                        n1663 = call "Set pump parameters.vi"("Pump write delay (ms)"=w2509, "Volume (uL)"="Ch 1 Inject Volume (uL)", "Rate (uL/h)"="Ch 1 Inject Rate (ul/h)", "Units"=4.0, "Pump #"=1.0, "Pump Parameters In"=w2515, "VISA resource name"=w2514) -> ("Pump Parameters Out"=w2507:T44)  [unwired: 3 in]
                        n1664 = Bundle By Name(cluster=w2508, "Pump 1"=w2507) -> (w2506:T7)
                        n1665 = local write "All Pump Parameters"(w2506) -> ()
                      }
                      frame #1 {
                        n1666 = Wait (ms)(milliseconds to wait=w2516) -> ()  [unwired: 1 out]
                      }
                      frame #2 {
                        n1667 = call "Write to pump.vi"("string"="start", "VISA resource name"=w2517) -> ()  [unwired: 1 out]
                      }
                      frame #3 {
                        n1668 = Wait (ms)(milliseconds to wait=u32 500) -> ()  [unwired: 1 out]
                      }
                      frame #4 {
                        n1669 = call "Write to pump.vi"("string"="start", "VISA resource name"=w2521) -> ()  [unwired: 1 out]
                      }
                    }
                  }
                }
              }
              frame True {
                n1670 = case shown="False" w2526 {
                  tunnel: w2527 -> [w2539 w2549]
                  frame False {
                    n1671 = flat-sequence {
                      tunnel: w2539 -> [w2541]
                      frame #0 {
                        n1672 = local write "Flushing P1"(FALSE ("Flushing P1")) -> ()
                        n1673 = Concatenate Strings("stop" ("string"), "\r") -> (w2543:string)
                        n1674 = VISA Write(VISA resource name=w2541, write buffer=w2543) -> ()  [unwired: 1 in, 3 out]
                      }
                      frame #1 {
                        n1675 = property on="Clear Volume P1" class="Bool (strict)"("Val(Sgnl)"=TRUE ("Value (Signaling)")) -> ()  [unwired: 2 in, 2 out]
                      }
                    }
                  }
                  frame True {
                    n1676 = local read "Normal Flow Rate (ul/h) P1"() -> (w2547:dbl)
                    n1677 = Number To Decimal String(number=w2547) -> (decimal integer string=w2553:string)  [unwired: 1 in]
                    n1678 = Concatenate Strings("irate  " ("string"), w2553, " u/h" ("string"), "\r") -> (w2551:string)
                    n1679 = VISA Write(VISA resource name=w2549, write buffer=w2551) -> (VISA resource name out=w2548:refnum<visa-resource-name>)  [unwired: 1 in, 2 out]
                    n1680 = Concatenate Strings("irun" ("string"), "\r") -> (w2555:string)
                    n1681 = VISA Write(VISA resource name=w2548, write buffer=w2555) -> ()  [unwired: 1 in, 3 out]
                  }
                }
                n1682 = local read "Saving..."() -> (w2524:bool)
                n1683 = local read "Save Event Log?"() -> (w2523:bool)
                n1684 = And(x=w2524, y=w2523) -> (x .and. y?=w2525:bool)
                n1685 = case shown="True" w2525 {
                  tunnel: w2526 -> [_ w2537]
                  frame False {
                  }
                  frame True {
                    n1686 = local read "Normal Flow Rate (ul/h) P1"() -> (w2528:dbl)
                    n1687 = Number To Decimal String(number=w2528) -> (decimal integer string=w2529:string)  [unwired: 1 in]
                    n1688 = Concatenate Strings("on, flow rate", w2529) -> (w2531:string)
                    n1689 = Select(t=w2531, s=w2537, f="off") -> (s? t:f=w2533:string)
                    n1690 = local read "log file ref"() -> (w2538:refnum<file>)
                    n1691 = local read "Time (s)"() -> (w2532:dbl)
                    n1692 = Concatenate Strings("pump 1 ", w2533) -> (w2535:string)
                    n1693 = call "write to event log.vi"("log file ref"=w2538, "time"=w2532, "input string"=w2535) -> ()  [unwired: 8 in]
                  }
                }
              }
            }
          }
          frame Enabled {
          }
        }
      }
      event "Inject Top:": Value Change {
        n1694 = event-data() -> ()  [unwired: 7 out]
        n1695 = call "hamilton_controller.vi"("Open?"="Inject Top:", "valve"=enum16{"A", "B", "C", "D", "ALL"}."A", "action"=T32."MOVE VALVE") -> ("error out"=w2557:errorcluster)  [unwired: 7 in, 1 out]
      }
      event "Inject Bottom:": Value Change {
        n1696 = event-data() -> ()  [unwired: 7 out]
        n1697 = call "hamilton_controller.vi"("Open?"="Inject Bottom:", "valve"=enum16{"A", "B", "C", "D", "ALL"}."B", "action"=T32."MOVE VALVE") -> ("error out"=w2561:errorcluster)  [unwired: 7 in, 1 out]
      }
      event "Inject Main:": Value Change {
        n1698 = event-data() -> ()  [unwired: 7 out]
        n1699 = call "hamilton_controller.vi"("Open?"="Inject Main:", "valve"=enum16{"A", "B", "C", "D", "ALL"}."C", "action"=T32."MOVE VALVE") -> ("error out"=w2565:errorcluster)  [unwired: 7 in, 1 out]
      }
      event "Inject Pump 3": Value Change {
        n1700 = event-data() -> ()  [unwired: 7 out]
        n1701 = local read "Use Harvard pumps\nfor beads (else Chemyx)"() -> (w2570:bool)
        n1702 = disable-structure shown="Disabled" {
          disable-tunnel: w2570 -> [w2572 _]
          disable-tunnel: w2569 -> [w2571 _]
          frame Disabled {
            n1703 = case shown="True" w2572 {
              tunnel: "Inject Pump 3" -> [w2576 w2617]
              tunnel: w2571 -> [_ w2618]
              frame False {
                n1704 = local read "Pump write delay (ms)"() -> (w2575:dbl)
                n1705 = case shown="True" w2576 {
                  tunnel: w2575 -> [w2582 w2596]
                  tunnel: "Chemyx Syringe Pump Serial Port" -> [w2579 w2595]
                  frame False {
                    n1706 = flat-sequence {
                      tunnel: w2579 -> [w2583]
                      tunnel: [w2583] -> w2580
                      tunnel: w2582 -> [_]
                      tunnel: [w2586] -> w2581
                      tunnel: w2580 -> [w2586]
                      tunnel: w2581 -> [w2587]
                      tunnel: [w2587] -> w2577
                      tunnel: [w2589] -> w2578
                      tunnel: w2577 -> [w2589]
                      tunnel: w2578 -> [w2591]
                      frame #0 {
                        n1707 = call "Write to pump.vi"("string"="enter pump3", "VISA resource name"=w2583) -> ()  [unwired: 1 out]
                      }
                      frame #1 {
                        n1708 = local read "Pump pause delay (ms)"() -> (w2585:u32)
                        n1709 = Wait (ms)(milliseconds to wait=w2585) -> ()  [unwired: 1 out]
                      }
                      frame #2 {
                        n1710 = call "Write to pump.vi"("string"="stop", "VISA resource name"=w2587) -> ()  [unwired: 1 out]
                      }
                      frame #3 {
                        n1711 = Wait (ms)(milliseconds to wait=u32 0) -> ()  [unwired: 1 out]
                      }
                      frame #4 {
                        n1712 = call "Write to pump.vi"("string"="stop", "VISA resource name"=w2591) -> ()  [unwired: 1 out]
                      }
                    }
                  }
                  frame True {
                    n1713 = flat-sequence {
                      tunnel: w2595 -> [w2605]
                      tunnel: w2596 -> [w2600]
                      tunnel: w2596 -> [w2607]
                      tunnel: w2595 -> [w2608]
                      tunnel: [w2608] -> w2594
                      tunnel: [w2611] -> w2593
                      tunnel: w2594 -> [w2611]
                      tunnel: w2593 -> [w2612]
                      frame #0 {
                        n1714 = local read "All Pump Parameters"() -> (w2599:T7)
                        n1715 = Unbundle By Name(w2599) -> ("Pump 3"=w2606:T44)
                        n1716 = call "Set pump parameters.vi"("Pump write delay (ms)"=w2600, "Volume (uL)"="Ch 3 Inject Volume (uL)", "Rate (uL/h)"="Ch 3 Inject Rate (ul/h)", "Units"=4.0, "Pump #"=3.0, "Pump Parameters In"=w2606, "VISA resource name"=w2605) -> ("Pump Parameters Out"=w2598:T44)  [unwired: 3 in]
                        n1717 = Bundle By Name(cluster=w2599, "Pump 3"=w2598) -> (w2597:T7)
                        n1718 = local write "All Pump Parameters"(w2597) -> ()
                      }
                      frame #1 {
                        n1719 = Wait (ms)(milliseconds to wait=w2607) -> ()  [unwired: 1 out]
                      }
                      frame #2 {
                        n1720 = call "Write to pump.vi"("string"="start", "VISA resource name"=w2608) -> ()  [unwired: 1 out]
                      }
                      frame #3 {
                        n1721 = Wait (ms)(milliseconds to wait=u32 500) -> ()  [unwired: 1 out]
                      }
                      frame #4 {
                        n1722 = call "Write to pump.vi"("string"="start", "VISA resource name"=w2612) -> ()  [unwired: 1 out]
                      }
                    }
                  }
                }
              }
              frame True {
                n1723 = case shown="False" w2617 {
                  tunnel: w2618 -> [w2630 w2637]
                  frame False {
                    n1724 = flat-sequence {
                      tunnel: w2630 -> [w2632]
                      frame #0 {
                        n1725 = local write "Flushing P3"(FALSE ("Flushing P3")) -> ()
                        n1726 = Concatenate Strings("stop" ("string"), "\r") -> (w2634:string)
                        n1727 = VISA Write(VISA resource name=w2632, write buffer=w2634) -> ()  [unwired: 1 in, 3 out]
                      }
                      frame #1 {
                        n1728 = property on="Clear Volume P3" class="Bool (strict)"("Val(Sgnl)"=TRUE ("Value (Signaling)")) -> ()  [unwired: 2 in, 2 out]
                      }
                    }
                  }
                  frame True {
                    n1729 = local read "Normal Flow Rate (ul/h) P3"() -> (w2638:dbl)
                    n1730 = Number To Decimal String(number=w2638) -> (decimal integer string=w2644:string)  [unwired: 1 in]
                    n1731 = Concatenate Strings("irate  " ("string"), w2644, " u/h" ("string"), "\r") -> (w2642:string)
                    n1732 = VISA Write(VISA resource name=w2637, write buffer=w2642) -> (VISA resource name out=w2640:refnum<visa-resource-name>)  [unwired: 1 in, 2 out]
                    n1733 = Concatenate Strings("irun" ("string"), "\r") -> (w2646:string)
                    n1734 = VISA Write(VISA resource name=w2640, write buffer=w2646) -> ()  [unwired: 1 in, 3 out]
                  }
                }
                n1735 = local read "Save Event Log?"() -> (w2615:bool)
                n1736 = local read "Saving..."() -> (w2616:bool)
                n1737 = And(x=w2616, y=w2615) -> (x .and. y?=w2614:bool)
                n1738 = case shown="True" w2614 {
                  tunnel: w2617 -> [_ w2625]
                  frame False {
                  }
                  frame True {
                    n1739 = local read "Normal Flow Rate (ul/h) P3"() -> (w2619:dbl)
                    n1740 = Number To Decimal String(number=w2619) -> (decimal integer string=w2621:string)  [unwired: 1 in]
                    n1741 = Concatenate Strings("on, flow rate", w2621) -> (w2620:string)
                    n1742 = local read "log file ref"() -> (w2624:refnum<file>)
                    n1743 = Select(t=w2620, s=w2625, f="off") -> (s? t:f=w2626:string)
                    n1744 = local read "Time (s)"() -> (w2623:dbl)
                    n1745 = Concatenate Strings("pump 3 ", w2626) -> (w2628:string)
                    n1746 = call "write to event log.vi"("log file ref"=w2624, "time"=w2623, "input string"=w2628) -> ()  [unwired: 8 in]
                  }
                }
              }
            }
          }
          frame Enabled {
          }
        }
      }
      event "Inject Pump 2": Value Change {
        n1747 = event-data() -> ()  [unwired: 7 out]
        n1748 = local read "Pump write delay (ms)"() -> (w2653:dbl)
        n1749 = flat-sequence {
          tunnel: w2652 -> [w2677]
          tunnel: w2653 -> [w2673]
          tunnel: "Inject Pump 2" -> [_]
          tunnel: w2653 -> [w2679]
          tunnel: w2652 -> [w2680]
          frame #0 {
            n1750 = local read "All Pump Parameters"() -> (w2672:T7)
            n1751 = Multiply(x=60.0, y="Flush Center Ch Rate (ul/m)") -> (x*y=w2669:dbl)
            n1752 = Unbundle By Name(w2672) -> ("Pump 2"=w2678:T44)
            n1753 = call "Set pump parameters.vi"("Pump write delay (ms)"=w2673, "Volume (uL)"="Flush Center Ch Volume (uL)", "Rate (uL/h)"=w2669, "Units"=3.0, "Pump #"=2.0, "Pump Parameters In"=w2678, "VISA resource name"=w2677) -> ("Pump Parameters Out"=w2671:T44)  [unwired: 3 in]
            n1754 = Bundle By Name(cluster=w2672, "Pump 2"=w2671) -> (w2670:T7)
            n1755 = local write "All Pump Parameters"(w2670) -> ()
            n1756 = Add(x="Flush Center Ch Volume (uL)", y="Total Volume\nFlushed (uL)") -> (x+y=w2666:dbl)
            n1757 = local write "Total Volume\nFlushed (uL)"(w2666) -> ()
          }
          frame #1 {
            n1758 = Wait (ms)(milliseconds to wait=w2679) -> ()  [unwired: 1 out]
          }
          frame #2 {
            n1759 = call "Write to pump.vi"("string"="start", "VISA resource name"=w2680) -> ()  [unwired: 1 out]
          }
        }
        n1760 = local read "Chemyx Syringe Pump Serial Port"() -> (w2652:refnum<visa-resource-name>)
        n1761 = local read "Save Event Log?"() -> (w2651:bool)
        n1762 = local read "Saving..."() -> (w2650:bool)
        n1763 = And(x=w2651, y=w2650) -> (x .and. y?=w2649:bool)
        n1764 = case shown="True" w2649 {
